vi "PurePursuitWithVision.vi"(6 "Gains":T4={"FFV"=0.0061, "FFA"=0.0025, "Vel PID"={"P"=0.01, "I"=0.0, "D"=0.0}} {"Vel PID"."D" format="%.3f"; "Vel PID"."I" format="%.3f"; "Vel PID"."P" format="%.3f"}, 8 "Reset":bool, 9 "UseVision":bool=TRUE, 10 "RobotNeededPathData":T2={"Path"=[{180.63328822733422, 252.5358592692828}, {179.0638472686962, 257.08345209094244}, {177.44994279683362, 261.5786143760306}, {175.74544648188558, 265.9669847301192}, {173.90094716897482, 270.19034998702415}, {171.861958652826, 274.1844888834733}, {169.56689181363876, 277.8768089203733}, {166.94484933881793, 281.1837519684998}, {163.913082773689, 284.0077834752845}, {160.36908573444177, 286.3182975096535}, {156.40209341301255, 288.2043413724174}, {152.08593998703844, 289.73951475940396}, {147.4817701115236, 290.98466483874887}, {142.6402774876305, 291.9901070067957}, {137.60353932715853, 292.7974469761464}, {132.40652884099228, 293.44108320885823}, {127.07837912520749, 293.9494551872971}, {121.6434480279992, 294.3460823917287}, {116.12221386609657, 294.65042476652826}, {110.53202506150767, 294.87859112011256}, {104.88772853519633, 295.0439218584949}, {99.20220360534157, 295.15747082323855}, {93.48682621065156, 295.22840631968967}, {87.751880335918, 295.2643459351343}, {82.00694325812172, 295.2716345397634}, {76.26120607621574, 295.2555804776057}, {70.52388786260789, 295.22063118252345}, {64.80442935368976, 295.1705811616298}, {59.113010594460434, 295.108618396024}, {53.46079936776458, 295.0375647699604}, {47.86035696817554, 294.9598768517579}, {42.326164867016196, 294.87775956345695}, {36.875125255569856, 294.7932844468561}, {31.52713045935557, 294.70843836467867}, {26.305818673883625, 294.6251691474966}], "MaxVel"=60.0, "MaxAccel"=40.0, "Backwards?"=FALSE, "PointSpacing"=6.0, "LookaheadDist"=16.0, "Speed/Curve"=2.0, "SlowDistanceAtEnd"=0.0, "SlowSpeed"=0.0, "MaxDeAccel"=40.0} {"SlowSpeed" format="%#_13g"; "SlowDistanceAtEnd" format="%#_13g"; "Speed/Curve" format="%#_13g"}, 11 "SensorData":T3={"LeftDistance"=537.92262, "RightDistance"=717.21774, "LeftVelocity"=-5.589, "RightVelocity"=-3.7260000000000004, "Angle"=159.66000000000003, "Location"={31.137993806145538, 289.8710865198651}}) -> (0 "Done":bool, 2 "RightValue":dbl=0.22465946197509765, 3 "LeftValue":dbl=0.2753405380249023)   [LabVIEW 2018]
uses:
  Dawgma Programming Library/Controls/PurePursuit/RobotNeededPathData.ctl
  Configuration/Constants.vi
  Implementation/Drive Published Globals.vi
  <vilib>/Rock Robotics/Network Tables/NT Read Number.vi
  <vilib>/addons/control/pid/pid.llb/PID (DBL).vi
  <vilib>/addons/control/pid/NI_PID_pid.lvlib
panel:
  out "Waveform Chart":dbl(graph)=1.6893692016601562
  in  "PID gains":T1={"proportional gain (Kc)"=0.015, "integral time (Ti, min)"=0.0, "derivative time (Td, min)"=0.1} {"derivative time (Td, min)" format="%.5f"; "integral time (Ti, min)" format="%.3f"; "proportional gain (Kc)" format="%.3f"}
  in  "output range":cluster{"output high":dbl, "output low":dbl}={"output high"=0.4, "output low"=-0.4} {"output low" format="%.2f"; "output high" format="%.2f"}
  in  "Throttle":dbl=0.25
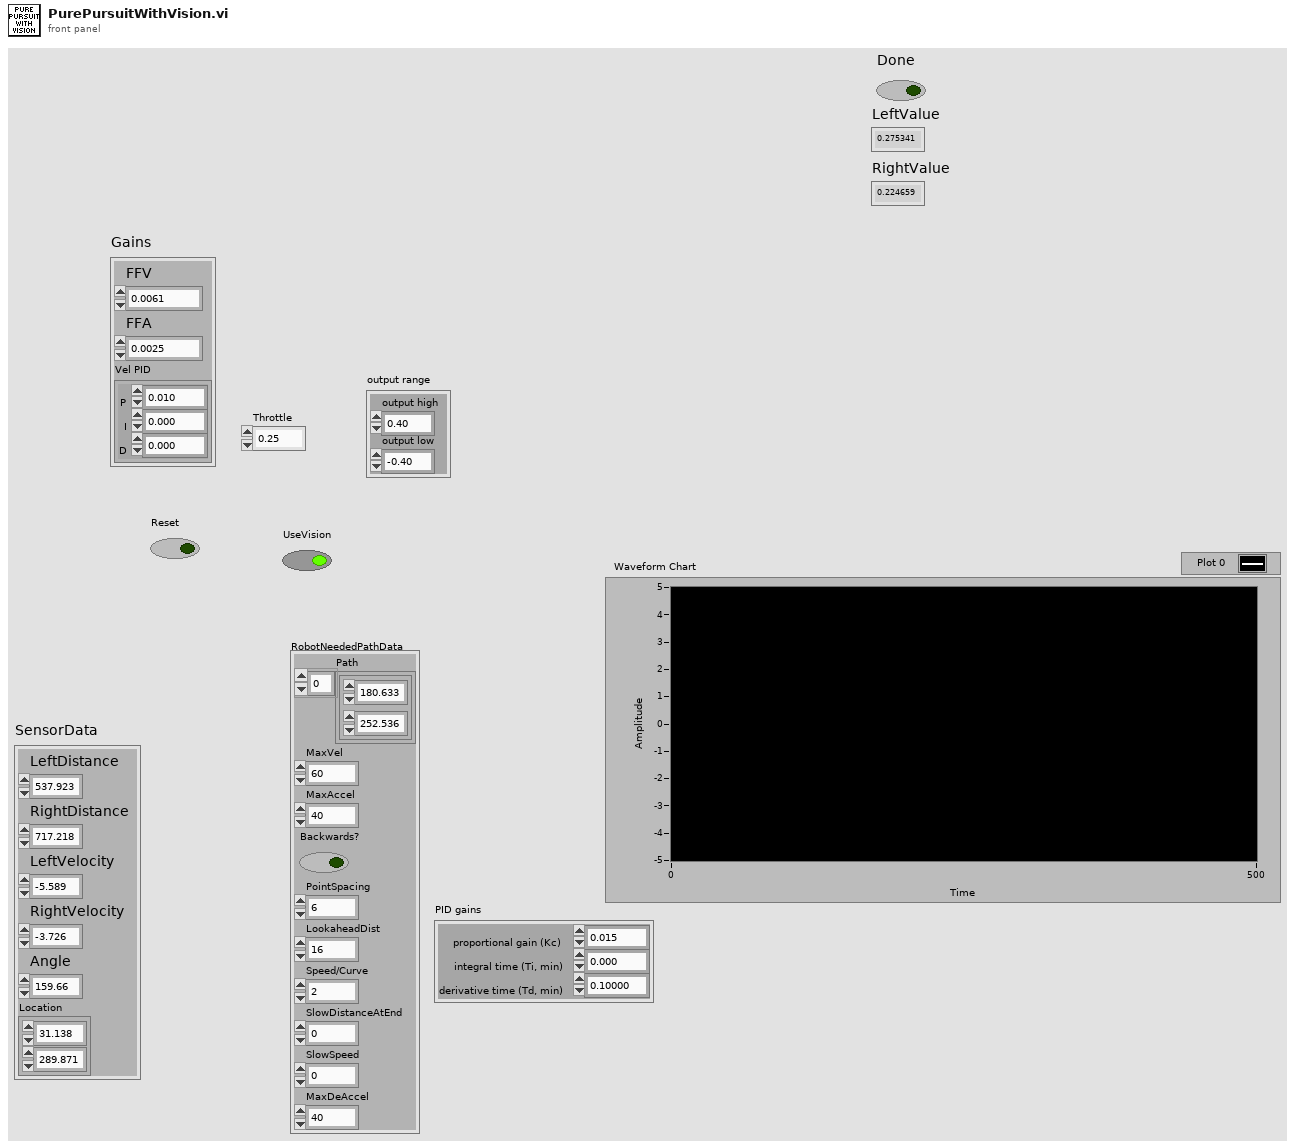
[diagram p1: front panel]
types:
  T1 = cluster{"proportional gain (Kc)":dbl, "integral time (Ti, min)":dbl, "derivative time (Td, min)":dbl}
  T2 = typedef "RobotNeededPathData.ctl" = cluster{"Path":cluster{dbl, dbl}[], "MaxVel":dbl, "MaxAccel":dbl, "Backwards?":bool, "PointSpacing":dbl, "LookaheadDist":dbl, "Speed/Curve":dbl, "SlowDistanceAtEnd":dbl, "SlowSpeed":dbl, "MaxDeAccel":dbl}
  T3 = cluster{"LeftDistance":dbl, "RightDistance":dbl, "LeftVelocity":dbl, "RightVelocity":dbl, "Angle":dbl, "Location":cluster{dbl, dbl}}
  T4 = cluster{"FFV":dbl, "FFA":dbl, "Vel PID":cluster{"P":dbl, "I":dbl, "D":dbl}}
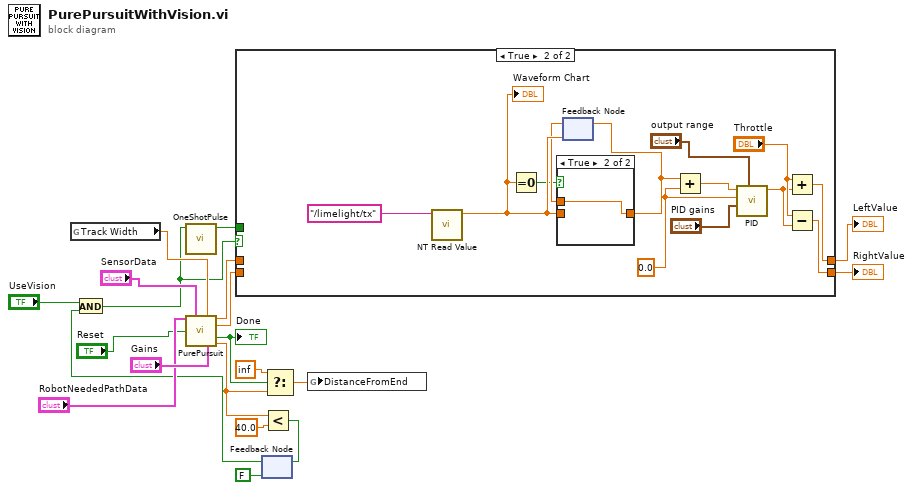
[diagram p0: block diagram]
diagram:
  n1 = global read "Constants.vi" "Track Width"() -> (w20:dbl)
  n2 = call "PurePursuit.vi"("RobotNeededPathData"="RobotNeededPathData", "SensorData"="SensorData", "Trackwidth"=w20, "Reset"="Reset", "Gains"="Gains") -> ("LeftValue"=w6:dbl, "RightValue"=w5:dbl, "Done"=w12:bool, "DistanceToEnd"=w17:dbl)  [unwired: 5 in, 2 out]
  "Done" <- w12
  n3 = feedback #1(FALSE) -> (w9:bool)
  n4 = And(x="UseVision", y=w9) -> (x .and. y?=w1:bool)
  n5 = call "OneShotPulse.vi"("Input"=w1) -> ("Output"=w2:bool)  [unwired: 10 in]
  n6 = case shown="True" w1 {
    tunnel: w6 -> [w22 _]
    tunnel: w5 -> [w21 _]
    tunnel: [w22 w25] -> w4
    tunnel: [w21 w24] -> w3
    tunnel: w2 -> [_ _]
    frame False {
    }
    frame True {
      w26 = 0.0 ("Gyro")
      n7 = call-poly <vilib>:"NT Read Value.vi"("Name"="/limelight/tx") -> ("Numeric"=w35:dbl)  [unwired: 9 in, 1 out]
      "Waveform Chart" <- w35
      n8 = Equal To 0?(x=w35) -> (x = 0?=w31:bool)
      n9 = feedback #2(w35) -> (w32:dbl)
      n10 = case shown="True" w31 {
        tunnel: w35 -> [w36 _]
        tunnel: [w36 w37] -> w33
        tunnel: w32 -> [_ w37]
        frame False {
        }
        frame True {
        }
      }
      n11 = feedback-in #2(w33) -> ()
      n12 = Add(x=w33, y=w26) -> (x+y=w34:dbl)
      n13 = call-poly <vilib>:"PID.vi"("output range"="output range", "PID gains"="PID gains", "process variable"=w26, "setpoint"=w34) -> ("output"=w23:dbl)  [unwired: 6 in, 1 out]
      n14 = Add(x="Throttle", y=w23) -> (x+y=w25:dbl)
      n15 = Subtract(x="Throttle", y=w23) -> (x-y=w24:dbl)
    }
  }
  "LeftValue" <- w4
  "RightValue" <- w3
  n16 = Less?(x=w17, y=40.0) -> (x < y?=w10:bool)
  n17 = feedback-in #1(w10) -> ()
  n18 = Select(t=inf, s=w12, f=w17) -> (s? t:f=w19:dbl)
  n19 = global write "Drive Published Globals.vi" "DistanceFromEnd"(w19) -> ()
